vi "Network Ping v2.0.vi"(0 "IP/Address":string="127.0.0.1", 5 "SetSize":i32=32, 7 "timeout":i32=100, 11 "error in (no error)":errorcluster) -> (4 "Status":i32(ring) items=["Success"=0, "DestinationNetworkUnreachable"=11002, "DestinationHostUnreachable"=11003, "DestinationProhibited, DestinationProtocolUnreachable"=11004, "DestinationPortUnreachable"=11005, "NoResources"=11006, "BadOption"=11007, "HardwareError"=11008, "PacketTooBig"=11009, "TimedOut"=11010, "BadRoute"=11012, "TtlExpired"=11013, "TtlReassemblyTimeExceeded"=11014, "ParameterProblem"=11015, "SourceQuench"=11016, "BadDestination"=11018, "DestinationUnreachable"=11040, "TimeExceeded"=11041, "BadHeader"=11042, "UnrecognizedNextHeader"=11043, "IcmpError"=11044, "DestinationScopeMismatch"=11045, "Unknown"=-1], 6 "RoundtripTime":i64, 8 "Ping OK?":bool, 15 "error out":errorcluster)   [LabVIEW 2020]
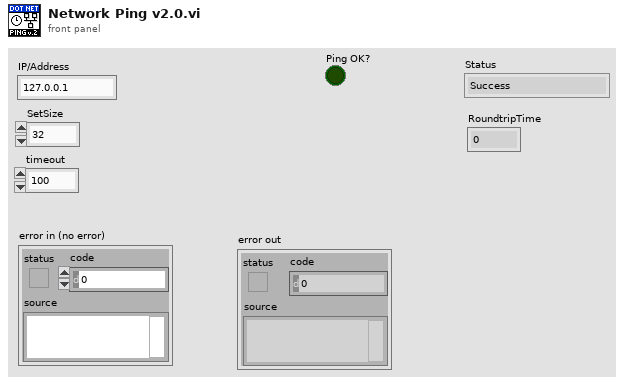
[diagram p1: front panel]
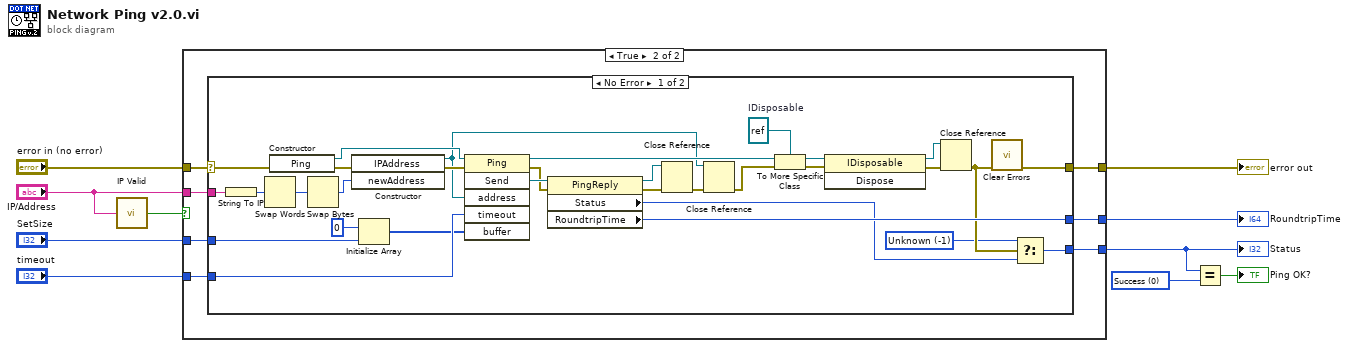
[diagram p0: block diagram]
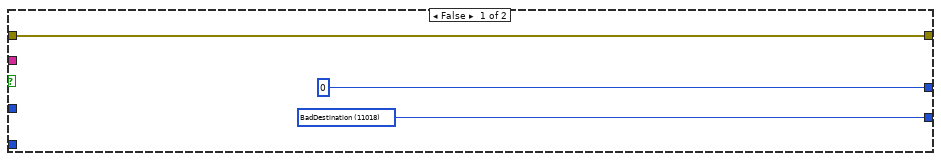
[diagram p2: hidden frame]
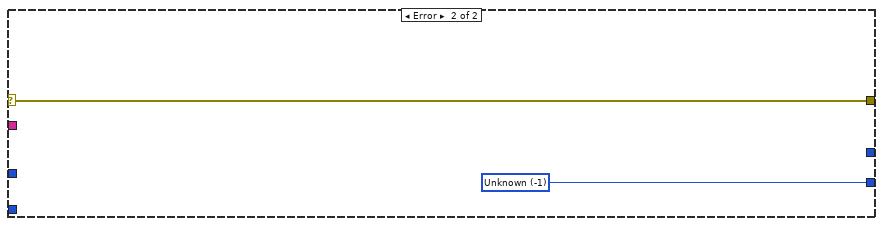
[diagram p3: hidden frame]
diagram:
  w2 = 0 items=["Success"=0, "DestinationNetworkUnreachable"=11002, "DestinationHostUnreachable"=11003, "DestinationProhibited, DestinationProtocolUnreachable"=11004, "DestinationPortUnreachable"=11005, "NoResources"=11006, "BadOption"=11007, "HardwareError"=11008, "PacketTooBig"=11009, "TimedOut"=11010, "BadRoute"=11012, "TtlExpired"=11013, "TtlReassemblyTimeExceeded"=11014, "ParameterProblem"=11015, "SourceQuench"=11016, "BadDestination"=11018, "DestinationUnreachable"=11040, "TimeExceeded"=11041, "BadHeader"=11042, "UnrecognizedNextHeader"=11043, "IcmpError"=11044, "DestinationScopeMismatch"=11045, "Unknown"=-1] ("Status")
  n1 = call "IP Valid.vi"("IP address"="IP/Address") -> ("Valid?"=w4:bool)
  n2 = case shown="True" w4 {
    tunnel: "timeout" -> [_ w20]
    tunnel: "SetSize" -> [_ w19]
    tunnel: [w12 w18] -> w3
    tunnel: [i64 0 ("RoundtripTime") w17] -> w8
    tunnel: [w13 w16] -> w7
    tunnel: "error in (no error)" -> [w13 w15]
    tunnel: "IP/Address" -> [_ w14]
    frame False {
      w12 = 11018 items=["Success"=0, "DestinationNetworkUnreachable"=11002, "DestinationHostUnreachable"=11003, "DestinationProhibited, DestinationProtocolUnreachable"=11004, "DestinationPortUnreachable"=11005, "NoResources"=11006, "BadOption"=11007, "HardwareError"=11008, "PacketTooBig"=11009, "TimedOut"=11010, "BadRoute"=11012, "TtlExpired"=11013, "TtlReassemblyTimeExceeded"=11014, "ParameterProblem"=11015, "SourceQuench"=11016, "BadDestination"=11018, "DestinationUnreachable"=11040, "TimeExceeded"=11041, "BadHeader"=11042, "UnrecognizedNextHeader"=11043, "IcmpError"=11044, "DestinationScopeMismatch"=11045, "Unknown"=-1] ("Status")
    }
    frame True {
      n3 = case shown="No Error" w15 {
        selector: w15 -> [w25 w53]
        tunnel: w14 -> [w51 _]
        tunnel: w20 -> [w50 _]
        tunnel: w19 -> [w49 _]
        tunnel: [w22 w52] -> w18
        tunnel: [w48 _] -> w17
        tunnel: [w47 w53] -> w16
        frame No Error {
          w21 = -1 items=["Success"=0, "DestinationNetworkUnreachable"=11002, "DestinationHostUnreachable"=11003, "DestinationProhibited, DestinationProtocolUnreachable"=11004, "DestinationPortUnreachable"=11005, "NoResources"=11006, "BadOption"=11007, "HardwareError"=11008, "PacketTooBig"=11009, "TimedOut"=11010, "BadRoute"=11012, "TtlExpired"=11013, "TtlReassemblyTimeExceeded"=11014, "ParameterProblem"=11015, "SourceQuench"=11016, "BadDestination"=11018, "DestinationUnreachable"=11040, "TimeExceeded"=11041, "BadHeader"=11042, "UnrecognizedNextHeader"=11043, "IcmpError"=11044, "DestinationScopeMismatch"=11045, "Unknown"=-1] ("Status")
          w35 = refnum<k24> refnum  # IDisposable
          n4 = String To IP(1:w51) -> (0:w39:u32)
          n5 = Swap Words(1:w39) -> (0:w37:u32)
          n6 = constructor class="Ping"(error in=w25) -> (reference out=w44:refnum<k24>, error out=w41:errorcluster)  [unwired: 2 in, 1 out]
          n7 = Swap Bytes(anything=w37) -> (byte swapped=w38:u32)
          n8 = constructor class="IPAddress"(error in=w41, "newAddress"=w38) -> (reference out=w31:refnum<k24>, error out=w40:errorcluster)  [unwired: 2 in, 2 out]
          n9 = Initialize Array(u8 0, w49) -> (w43:u8[])
          n10 = invoke class="Ping" method="Send"(reference=w44, error in=w40, "address"=w31, "timeout"=w50, "buffer"=w43) -> (reference out=w36:refnum<k24>, error out=w45:errorcluster, "Send"=w46:refnum<k24>)  [unwired: 1 in, 3 out]
          n11 = property class="PingReply"(reference=w46, error in=w45) -> (reference out=w34:refnum<k24>, error out=w33:errorcluster, "Status"=w23:i32, "RoundtripTime"=w48:i64)
          n12 = Close Reference(reference=w34, error in (no error)=w33) -> (error out=w32:errorcluster)
          n13 = Close Reference(reference=w31, error in (no error)=w32) -> (error out=w30:errorcluster)
          n14 = To More Specific Class(target class=w35, reference=w36, error in=w30) -> (specific class reference=w29:refnum<k24>, error out=w28:errorcluster)
          n15 = invoke class="IDisposable" method="Dispose"(reference=w29, error in=w28) -> (reference out=w26:refnum<k24>, error out=w27:errorcluster)  [unwired: 1 in, 1 out]
          n16 = Close Reference(reference=w26, error in (no error)=w27) -> (error out=w24:errorcluster)
          n17 = call <vilib>:"Clear Errors.vi"("error in (no error)"=w24) -> ("error out"=w47:errorcluster)  [unwired: 5 in, 1 out]
          n18 = Select(t=w21, s=w24, f=w23) -> (s? t:f=w22:i32)
        }
        frame Error {
          w52 = -1 items=["Success"=0, "DestinationNetworkUnreachable"=11002, "DestinationHostUnreachable"=11003, "DestinationProhibited, DestinationProtocolUnreachable"=11004, "DestinationPortUnreachable"=11005, "NoResources"=11006, "BadOption"=11007, "HardwareError"=11008, "PacketTooBig"=11009, "TimedOut"=11010, "BadRoute"=11012, "TtlExpired"=11013, "TtlReassemblyTimeExceeded"=11014, "ParameterProblem"=11015, "SourceQuench"=11016, "BadDestination"=11018, "DestinationUnreachable"=11040, "TimeExceeded"=11041, "BadHeader"=11042, "UnrecognizedNextHeader"=11043, "IcmpError"=11044, "DestinationScopeMismatch"=11045, "Unknown"=-1] ("Status")
        }
      }
    }
  }
  "RoundtripTime" <- w8
  "error out" <- w7
  "Status" <- w3
  n19 = Equal?(x=w3, y=w2) -> (x = y?=→"Ping OK?":bool)
